vi "Dynamic Scrollbars - Display.vi"(8 "error in":errorcluster, 10 "Active Display in":u16, 11 "VI Ref":refnum<vi>) -> (0 "error out":errorcluster, 2 "Active Display out":u16, 3 "VI Ref":refnum<vi>)   [LabVIEW 2014]
doc: "Makes horizontal and vertical scrollbars for every pane of the FP on/off depending on the size of the FP and the selected display.\n\nIt places the FP in the top left corner of the display."
uses:
  <vilib>/Utility/miscctls.llb/LVRectTypeDef.ctl
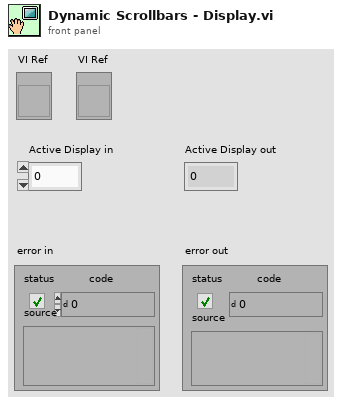
[diagram p1: front panel]
types:
  T1 = typedef "LVRectTypeDef.ctl" = cluster{"Left":i16, "Top":i16, "Right":i16, "Bottom":i16}
  T2 = cluster{"Left":i16, "Top":i16, "Right":i16, "Bottom":i16}
  T3 = enum16{"Always On", "Always Off", "Off While Running"}
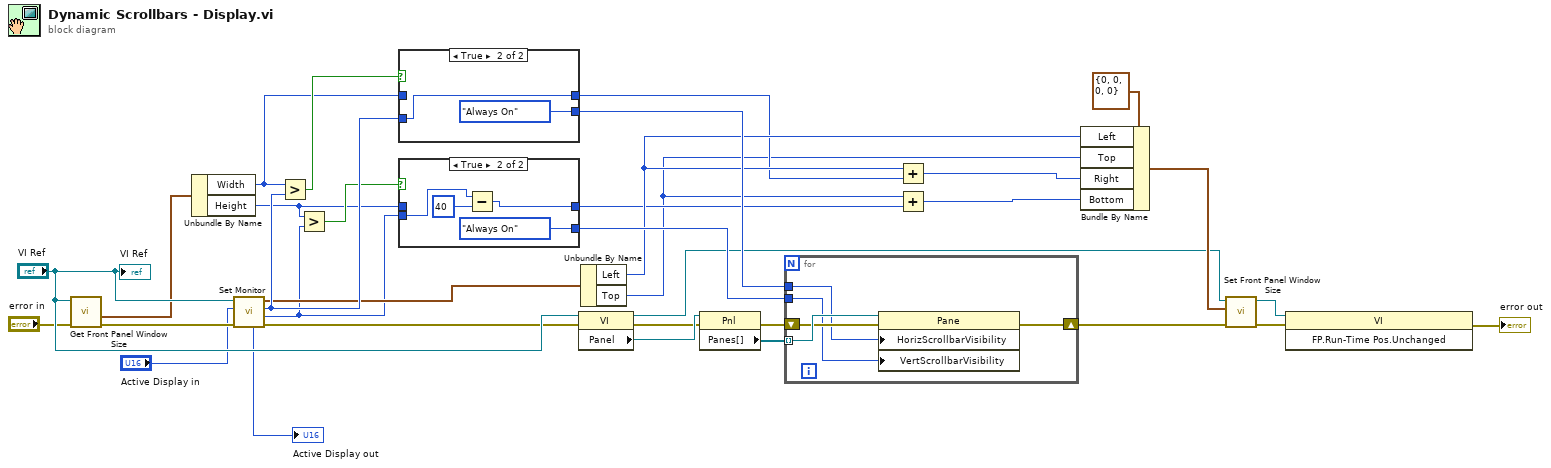
[diagram p0: block diagram]
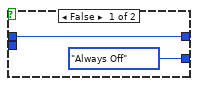
[diagram p2: hidden frame]
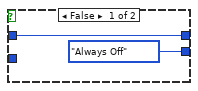
[diagram p3: hidden frame]
diagram:
  n1 = call "Get Front Panel Window Size.vi"("error in"="error in", "VI Ref"="VI Ref") -> ("error out"=w25:errorcluster, "FP:Window Size"=w5:cluster{"Width":i16, "Height":i16})  [unwired: 4 in, 4 out]
  n2 = Unbundle By Name(w5) -> ("Width"=w15:i16, "Height"=w13:i16)
  n3 = call "Set Monitor.vi"("error in"=w25, "FP:Monitor"="Active Display in", "VI Ref"="VI Ref") -> ("error out"=w3:errorcluster, "Disp.Height"=w2:i16, "Disp.Width"=w22:i16, "Disp.Bounds"=w9:T2, "Active Display"=→"Active Display out":u16)  [unwired: 4 in]
  n4 = Greater?(x=w15, y=w22) -> (0:w23:bool)
  n5 = Greater?(x=w13, y=w2) -> (0:w14:bool)
  n6 = case shown="True" w23 {
    tunnel: [T3."Always Off" ("Horizontal Scrollbar Visibility") T3."Always On" ("Horizontal Scrollbar Visibility")] -> w29
    tunnel: w15 -> [w34 _]
    tunnel: w22 -> [_ w36]
    tunnel: [w34 w36] -> w7
    frame False {
    }
    frame True {
    }
  }
  n7 = case shown="True" w14 {
    tunnel: [T3."Always Off" ("Horizontal Scrollbar Visibility") T3."Always On" ("Horizontal Scrollbar Visibility")] -> w28
    tunnel: w13 -> [w38 _]
    tunnel: [w38 w40] -> w10
    tunnel: w2 -> [_ w41]
    frame False {
    }
    frame True {
      n8 = Subtract(x=w41, y=i16 40) -> (x-y=w40:i16)
    }
  }
  n9 = property class="VI"(reference="VI Ref", error in=w3) -> (reference out=w8:refnum<vi>, error out=w32:errorcluster, "Panel"=w33:refnum<vi>)
  n10 = Unbundle By Name(w9) -> ("Left"=w11:i16, "Top"=w6:i16)
  n11 = property class="Pnl"(reference=w33, error in=w32) -> (error out=w31:errorcluster, "Panes[]"=w30:refnum<vi>[])  [unwired: 1 out]
  n12 = for {
    shift-right: [w46] -> w18
    shift-left: w31 -> [w47]
    tunnel: w30 -> [w48] mode=indexing
    tunnel: w29 -> [w45]
    tunnel: w28 -> [w44]
    n13 = property class="Pane"(reference=w48, error in=w47, "HorizScrollbarVisibility"=w45, "VertScrollbarVisibility"=w44) -> (error out=w46:errorcluster)  [unwired: 1 out]
  }
  n14 = Add(x=w11, y=w7) -> (x+y=w12:i16)
  n15 = Add(x=w6, y=w10) -> (x+y=w1:i16)
  n16 = Bundle By Name(cluster=T1 {"Left"=0, "Top"=0, "Right"=0, "Bottom"=0} ("Front Panel Window:Window Bounds"), "Left"=w11, "Top"=w6, "Right"=w12, "Bottom"=w1) -> (w17:T1)
  n17 = call "Set Front Panel Window Size.vi"("error in"=w18, "Front Panel Window:Window Bounds"=w17, "VI Ref"=w8) -> ("error out"=w19:errorcluster, "VI Ref"=w16:refnum<vi>)  [unwired: 7 in]
  n18 = invoke class="VI" method="FP.Run-Time Pos.Unchanged"(reference=w16, error in=w19) -> (error out=→"error out":errorcluster)  [unwired: 1 in, 2 out]
  "VI Ref" <- "VI Ref"
